vi "form-seq-TRABS-IR-SD.vi"(2 "II channel":u16[][](array[numeric]), 3 "Number of aq":i32, 4 "I channel":u16[][](array[numeric])) -> (0 "II channel seq":cluster{"BG":i32[], "Ie":u32[], "I0":i32[]}[](array[cluster]), 1 "I channel seq":cluster{"BG":i32[], "Ie":i32[], "I0":i32[]}[](array[cluster]))   [LabVIEW 2015]
panel:
  out "Brut camera out":u16[](graph) caption="Data Values"
  out "Brut camera 1 in":u16[](graph) caption="Data Values"
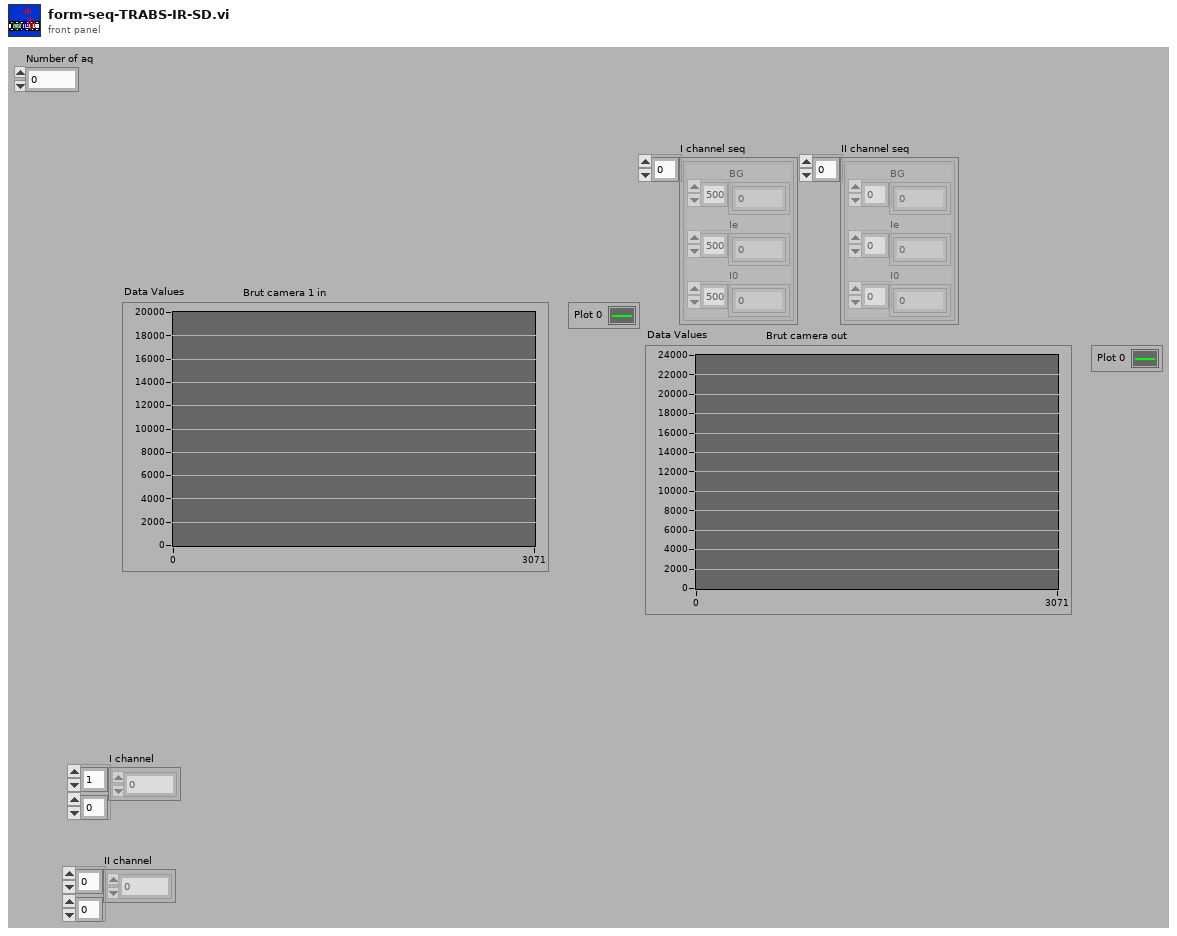
[diagram p1: front panel]
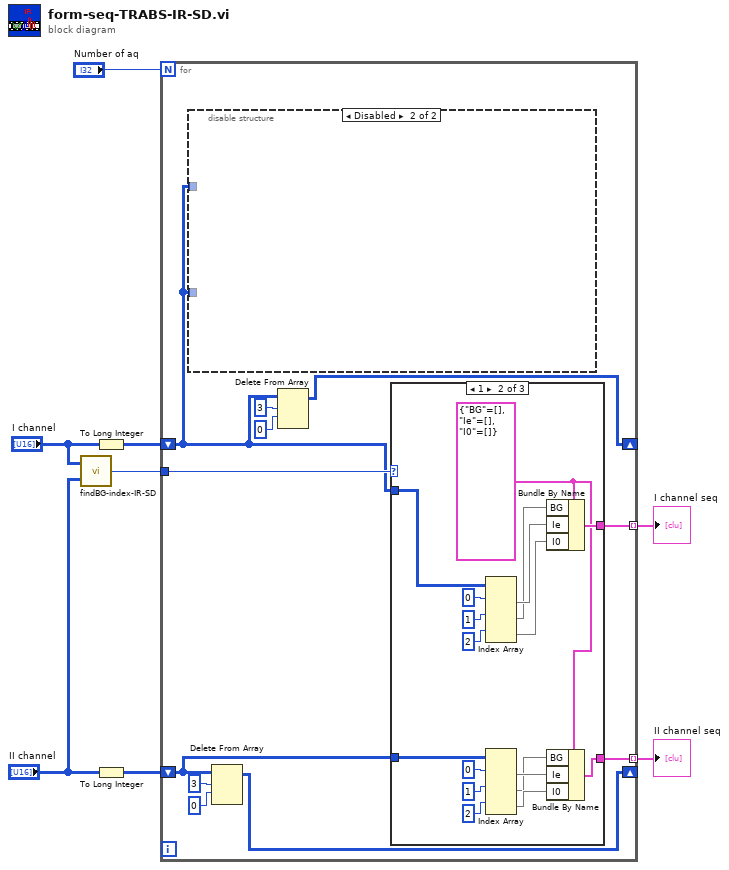
[diagram p0: block diagram]
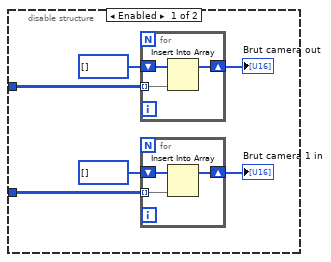
[diagram p2: hidden frame]
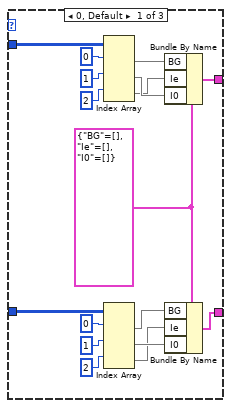
[diagram p3: hidden frame]
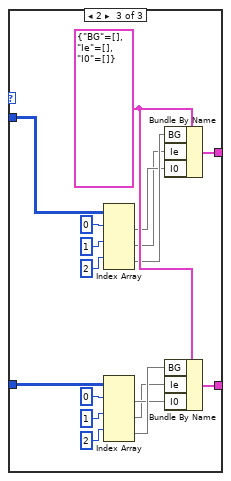
[diagram p4: hidden frame]
diagram:
  n1 = call "findBG-index-IR-SD.vi"("II channel in"="II channel", "I channel in"="I channel") -> ("index BG"=w2:i32)
  n2 = To Long Integer(number="I channel") -> (32bit integer=w5:i32[][])
  n3 = To Long Integer(number="II channel") -> (32bit integer=w6:i32[][])
  n4 = for {
    N: "Number of aq" -> [_]
    shift-right: [w14] -> _
    shift-left: w6 -> [w15]
    shift-right: [w11] -> _
    shift-left: w5 -> [w9]
    tunnel: [w13] -> w8 mode=indexing
    tunnel: [w12] -> w7 mode=indexing
    tunnel: w2 -> [w10]
    n5 = disable-structure shown="Disabled" {
      disable-tunnel: w9 -> [w25 _]
      disable-tunnel: w9 -> [w24 _]
      frame Enabled {
        n6 = for {
          tunnel: w24 -> [w27] mode=indexing
          shift-right: [w26] -> w21
          shift-left: u16[] [] ("I channel") -> [w28]
          n7 = Insert Into Array(array=w28, new element=w27) -> (w26:u16[])  [unwired: 1 in]
        }
        "Brut camera out" <- w21
        n8 = for {
          tunnel: w25 -> [w30] mode=indexing
          shift-right: [w29] -> w22
          shift-left: u16[] [] ("I channel") -> [w31]
          n9 = Insert Into Array(array=w31, new element=w30) -> (w29:u16[])  [unwired: 1 in]
        }
        "Brut camera 1 in" <- w22
      }
      frame Disabled {
      }
    }
    n10 = Delete From Array(array=w15, length=3 ("longueur"), index (row)=0 ("indice (ligne)")) -> (array with subset deleted=w14:i32[][])  [unwired: 1 in, 1 out]
    n11 = Delete From Array(array=w9, length=3 ("longueur"), index (row)=0 ("indice (ligne)")) -> (array with subset deleted=w11:i32[][])  [unwired: 1 in, 1 out]
    n12 = case shown="1" w10 {
      tunnel: w9 -> [w41 w49 w73]
      tunnel: w15 -> [w35 w56 w72]
      tunnel: [w40 w65 w82] -> w13
      tunnel: [w39 w64 w81] -> w12
      frame 0, Default {
        w45 = cluster{"BG":u16[], "Ie":u16[], "I0":u16[]} {"BG"=[], "Ie"=[], "I0"=[]} ("input cluster")
        n13 = Index Array(array=w41, index (row) #1=0 ("index (row)"), index (row) #2=1 ("index (row)"), index (row) #3=2 ("index (row)")) -> (element #1=w38:i32[], element #2=w37:i32[], element #3=w36:i32[])  [unwired: 3 in]
        n14 = Index Array(array=w35, index (row) #1=0 ("index (row)"), index (row) #2=1 ("index (row)"), index (row) #3=2 ("index (row)")) -> (element #1=w34:i32[], element #2=w33:i32[], element #3=w32:i32[])  [unwired: 3 in]
        n15 = Bundle By Name(cluster=w45, "BG"=w38, "Ie"=w36, "I0"=w37) -> (w40:cluster{"BG":u16[], "Ie":u16[], "I0":u16[]})
        n16 = Bundle By Name(cluster=w45, "BG"=w34, "Ie"=w32, "I0"=w33) -> (w39:cluster{"BG":u16[], "Ie":u16[], "I0":u16[]})
      }
      frame 1 {
        w60 = cluster{"BG":u16[], "Ie":u16[], "I0":u16[]} {"BG"=[], "Ie"=[], "I0"=[]} ("input cluster")
        n17 = Index Array(array=w49, index (row) #1=0 ("index (row)"), index (row) #2=1 ("index (row)"), index (row) #3=2 ("index (row)")) -> (element #1=w55:i32[], element #2=w53:i32[], element #3=w54:i32[])  [unwired: 3 in]
        n18 = Index Array(array=w56, index (row) #1=0 ("index (row)"), index (row) #2=1 ("index (row)"), index (row) #3=2 ("index (row)")) -> (element #1=w52:i32[], element #2=w50:i32[], element #3=w51:i32[])  [unwired: 3 in]
        n19 = Bundle By Name(cluster=w60, "BG"=w53, "Ie"=w55, "I0"=w54) -> (w65:cluster{"BG":u16[], "Ie":u16[], "I0":u16[]})
        n20 = Bundle By Name(cluster=w60, "BG"=w50, "Ie"=w52, "I0"=w51) -> (w64:cluster{"BG":u16[], "Ie":u16[], "I0":u16[]})
      }
      frame 2 {
        w77 = cluster{"BG":u16[], "Ie":u16[], "I0":u16[]} {"BG"=[], "Ie"=[], "I0"=[]} ("input cluster")
        n21 = Index Array(array=w73, index (row) #1=0 ("index (row)"), index (row) #2=1 ("index (row)"), index (row) #3=2 ("index (row)")) -> (element #1=w69:i32[], element #2=w68:i32[], element #3=w70:i32[])  [unwired: 3 in]
        n22 = Index Array(array=w72, index (row) #1=0 ("index (row)"), index (row) #2=1 ("index (row)"), index (row) #3=2 ("index (row)")) -> (element #1=w67:i32[], element #2=w66:i32[], element #3=w71:i32[])  [unwired: 3 in]
        n23 = Bundle By Name(cluster=w77, "BG"=w70, "Ie"=w68, "I0"=w69) -> (w82:cluster{"BG":u16[], "Ie":u16[], "I0":u16[]})
        n24 = Bundle By Name(cluster=w77, "BG"=w71, "Ie"=w66, "I0"=w67) -> (w81:cluster{"BG":u16[], "Ie":u16[], "I0":u16[]})
      }
    }
  }
  "I channel seq" <- w8
  "II channel seq" <- w7
